vi "Configure Sweep Settling.vi"(0 "VISA resource name":refnum<visa-resource-name>, 1 "Algorithm Type (0: stlNone)":i32(ring) items=["stlNone", "stlExponential", "stlFlat", "stlAverage", "stlSequential"], 2 "Tolerance (0)":dbl, 5 "Settler Number (0)":i32, 7 "Delay (0s)":dbl, 9 "Threshold (0)":dbl, 11 "error in (no error)":errorcluster, 12 "Number Of Points (2)":i32=2) -> (4 "VISA resource name out":refnum<visa-resource-name>, 15 "error out":errorcluster)   [LabVIEW 2014, in "Stanford Research SR1.lvlib"]
doc: "Configures the attributes for the Sweep Settling."
uses:
  Stanford Research SR1.lvlib
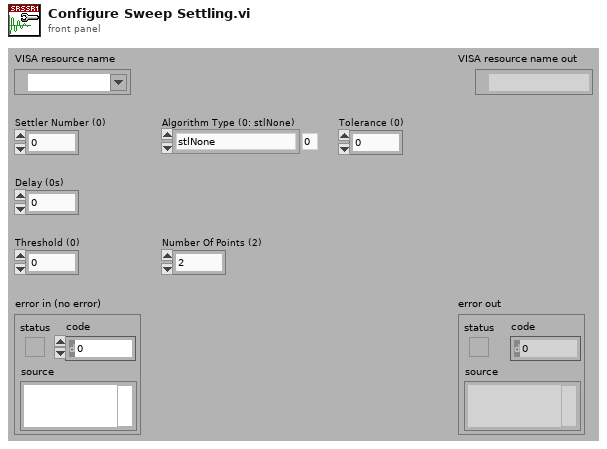
[diagram p1: front panel]
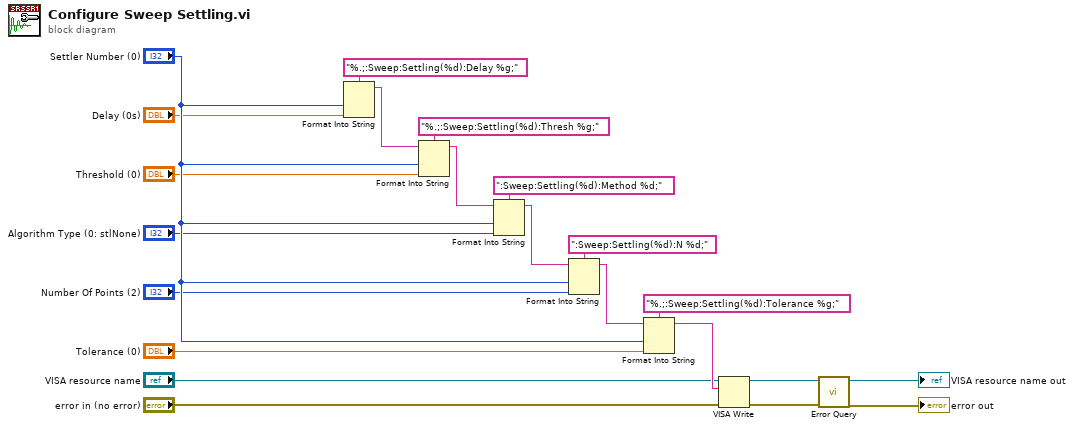
[diagram p0: block diagram]
diagram:
  n1 = Format Into String(format string="%.;:Sweep:Settling(%d):Delay %g;", "Settler Number (0)", "Delay (0s)") -> (resulting string=w21:string)  [unwired: 2 in, 1 out]
  n2 = Format Into String(format string="%.;:Sweep:Settling(%d):Thresh %g;", initial string=w21, "Settler Number (0)", "Threshold (0)") -> (resulting string=w19:string)  [unwired: 1 in, 1 out]
  n3 = Format Into String(format string=":Sweep:Settling(%d):Method %d;", initial string=w19, "Settler Number (0)", "Algorithm Type (0: stlNone)") -> (resulting string=w17:string)  [unwired: 1 in, 1 out]
  n4 = Format Into String(format string=":Sweep:Settling(%d):N %d;", initial string=w17, "Settler Number (0)", "Number Of Points (2)") -> (resulting string=w15:string)  [unwired: 1 in, 1 out]
  n5 = Format Into String(format string="%.;:Sweep:Settling(%d):Tolerance %g;", initial string=w15, "Settler Number (0)", "Tolerance (0)") -> (resulting string=w13:string)  [unwired: 1 in, 1 out]
  n6 = VISA Write(VISA resource name="VISA resource name", write buffer=w13, error in (no error)="error in (no error)") -> (VISA resource name out=w10:refnum<visa-resource-name>, error out=w9:errorcluster)  [unwired: 1 out]
  n7 = call "Error Query.vi"("error in (no error)"=w9, "VISA resource name"=w10) -> ("error out"=→"error out":errorcluster, "VISA resource name out"=→"VISA resource name out":refnum<visa-resource-name>)  [unwired: 6 in, 2 out]
